vi "mongo_cmd_drop_db.vi"(10 "db":string, 11 "conn":T1) -> (0 "result":errorcluster)   [LabVIEW 2013]
uses:
  mongo.ctl
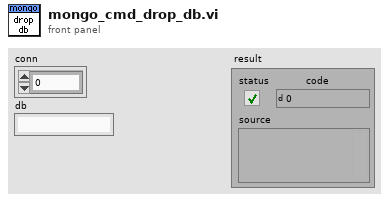
[diagram p1: front panel]
types:
  T1 = typedef "mongo.ctl" = cluster{i32}
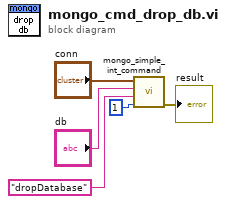
[diagram p0: block diagram]
diagram:
  n1 = call "mongo_simple_int_command.vi"("arg"=1, "cmdstr"="dropDatabase", "db"="db", "mongo"="conn") -> ("result"=→"result":errorcluster)  [unwired: 6 in, 1 out]
